vi "goToabsY.vi"(8 "error in":errorcluster, 11 "Y position":dbl) -> (0 "error out":errorcluster)   [LabVIEW 2014]
doc: "André Romero - 2023\nandretec@ifsc.usp.br\nIFSC - USP"
uses:
  Global Motors.vi
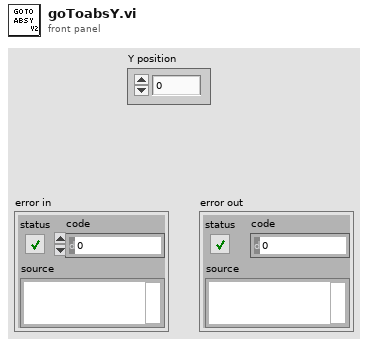
[diagram p1: front panel]
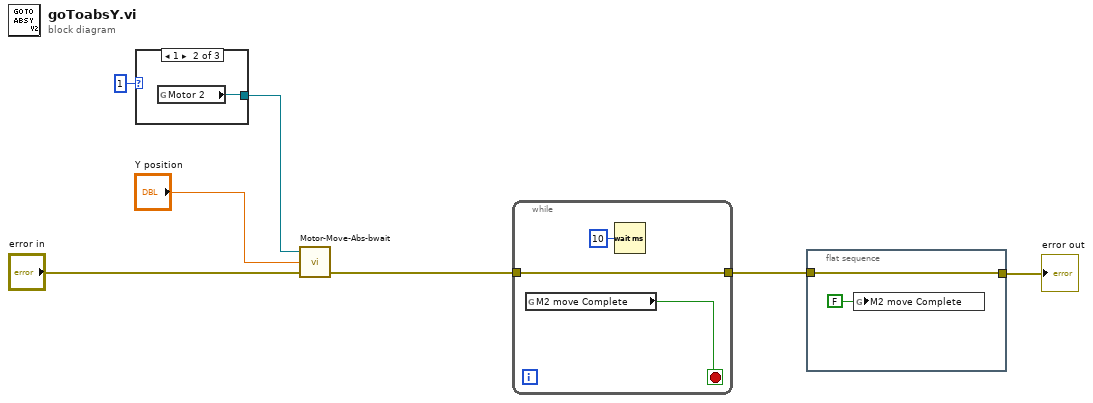
[diagram p0: block diagram]
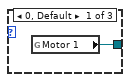
[diagram p2: hidden frame]
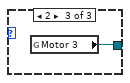
[diagram p3: hidden frame]
diagram:
  n1 = case shown="1" u16 1 ("Axis") {
    tunnel: [w8 w9 w10] -> w7
    frame 0, Default {
      n2 = global read "Global Motors.vi" "Motor 1"() -> (w8:refnum<k7>)
    }
    frame 1 {
      n3 = global read "Global Motors.vi" "Motor 2"() -> (w9:refnum<k7>)
    }
    frame 2 {
      n4 = global read "Global Motors.vi" "Motor 3"() -> (w10:refnum<k7>)
    }
  }
  n5 = call "Motor-Move-Abs-bwait.vi"("error"="error in", "Posição"="Y position", "MG17Motor A"=w7) -> ("error out"=w1:errorcluster)  [unwired: 1 in, 1 out]
  n6 = while {
    tunnel: w1 -> [w13]
    tunnel: [w13] -> w2
    stop <- w11 stop-if-true
    n7 = global read "Global Motors.vi" "M2 move Complete"() -> (w11:bool)
    n8 = Wait (ms)(milliseconds to wait=u32 10) -> ()  [unwired: 1 out]
  }
  n9 = flat-sequence {
    tunnel: w2 -> [w15]
    tunnel: [w15] -> w6
    frame #0 {
      n10 = global write "Global Motors.vi" "M2 move Complete"(FALSE ("M1 move Complete")) -> ()
    }
  }
  "error out" <- w6
